vi "FGV_StepMem.vi"(6 "Func":enum16{"Set", "Get"}(ring), 8 "StepE":i32) -> (0 "StepMem Out":i32)   [LabVIEW 2017]
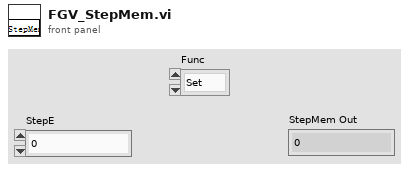
[diagram p1: front panel]
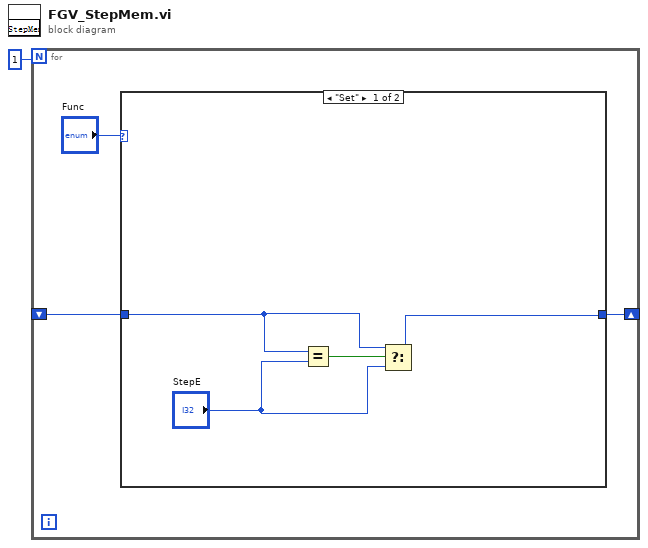
[diagram p0: block diagram]
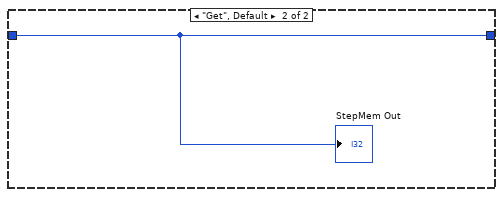
[diagram p2: hidden frame]
diagram:
  n1 = for {
    N: 1 -> [_]
    shift-right: [w3] -> _
    shift-left: _ -> [w2]
    n2 = case shown="\"Set\"" "Func" {
      tunnel: [w7 w9] -> w3
      tunnel: w2 -> [w5 w9]
      frame "Set" {
        n3 = Equal?(x=w5, y="StepE") -> (x = y?=w6:bool)
        n4 = Select(t=w5, s=w6, f="StepE") -> (s? t:f=w7:i32)
      }
      frame "Get", Default {
        "StepMem Out" <- w9
      }
    }
  }
